vi "Measure Current through  Charger Load.vi"(9 "DMM Voltages":dbl[](array[numeric]), 10 "R1 (Ohms)":dbl=2.0 step=0.1) -> (3 "Current (mA)":dbl format="%0.8f")   [LabVIEW 2015]
doc: "Mearsure the voltage on both sides of the resistor and divide by the resistance of the Load Resistor\nThis needs to be measured durring Fixture CAL procedure and entered into the config file"
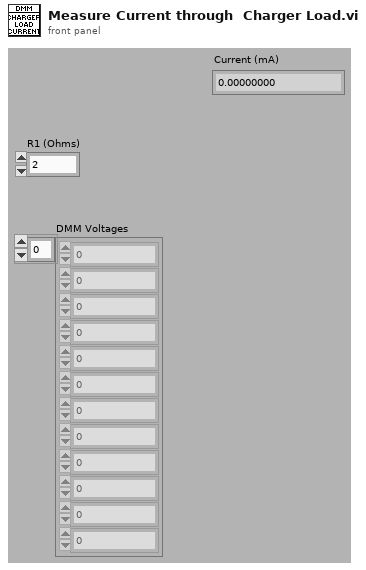
[diagram p1: front panel]
types:
  T1 = enum16{"Green LED 1", "Red LED", "VCELL", "VP2 TESTER", "TEMP TESTER", "Green LED 2"}
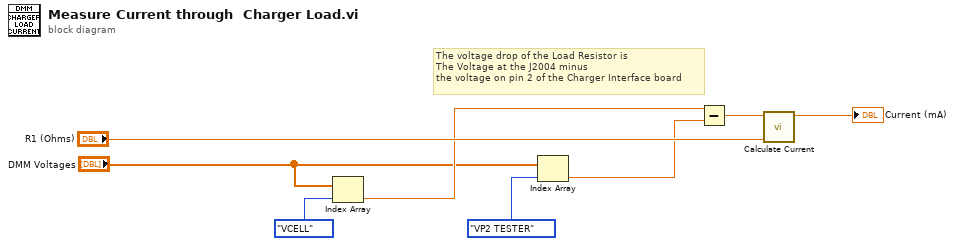
[diagram p0: block diagram]
diagram:
  # "The voltage drop of the Load Resistor is\nThe Voltage at the J2004 minus \nthe voltage on pin 2 of the Charger Interface board"
  n1 = Index Array(array="DMM Voltages", index=T1."VCELL" ("Selector")) -> (element=w5:dbl)
  n2 = Index Array(array="DMM Voltages", index=T1."VP2 TESTER" ("Selector")) -> (element=w4:dbl)
  n3 = Subtract(x=w5, y=w4) -> (x-y=w7:dbl)
  n4 = call "Calculate Current.vi"("R1 (Ohms)"="R1 (Ohms)", "Voltage Drop over Load (Volts)"=w7) -> ("Current (mA)"=→"Current (mA)":dbl)  [unwired: 9 in]
